vi "Rename Category.vi"(8 "error in (no error)":errorcluster, 9 "New Name":string, 10 "Old Name":string, 11 "Budgetizer in":refnum<class "Budgetizer.lvclass">) -> (0 "error out":errorcluster, 2 "Anything Renamed?":bool, 3 "Budgetizer out":refnum<class "Budgetizer.lvclass">)   [LabVIEW 2018, in "Budgetizer.lvclass"]
uses:
  Budgetizer.lvclass
  Budgetizer.lvclass/Budgetizer.ctl
  database/Database.lvclass
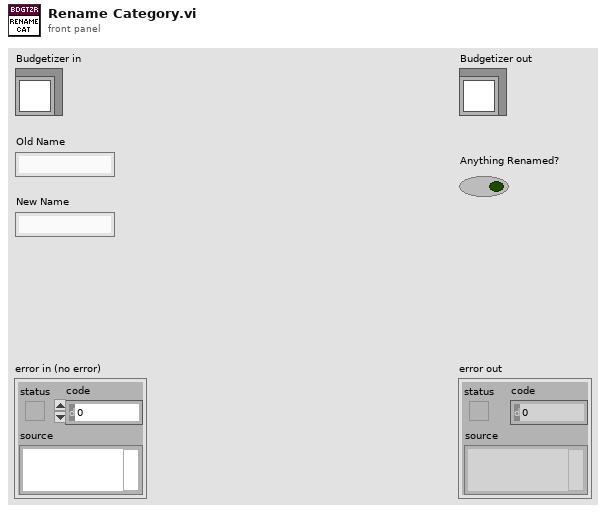
[diagram p1: front panel]
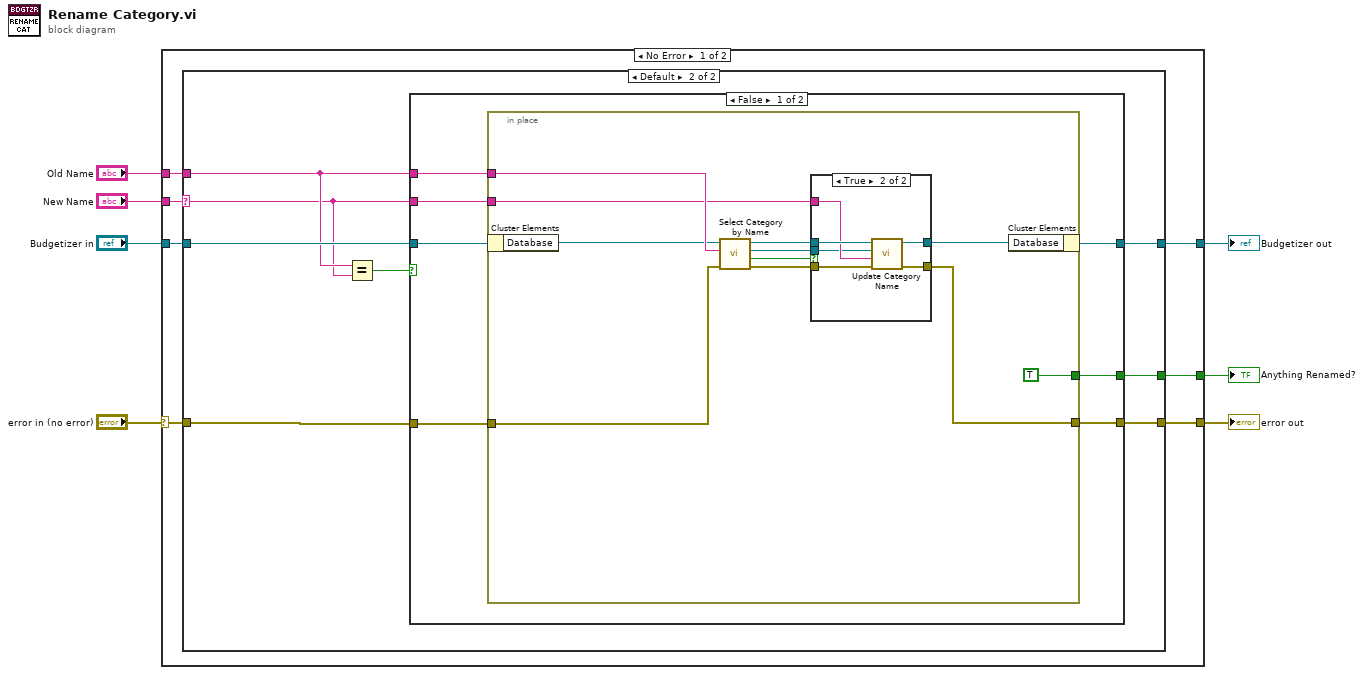
[diagram p0: block diagram]
diagram:
  n1 = case shown="No Error" "error in (no error)" {
    selector: "error in (no error)" -> [w9 w54]
    tunnel: [w8 w54] -> w6
    tunnel: [w10 w53] -> w4
    tunnel: "Budgetizer in" -> [w12 w53]
    tunnel: "Old Name" -> [w14 _]
    tunnel: "New Name" -> [w11 _]
    tunnel: [w13 _] -> w1
    frame No Error {
      n2 = case shown="Default" w11 {
        selector: w11 -> [_ w18]
        tunnel: w14 -> [_ w19]
        tunnel: [_ w20] -> w13
        tunnel: w12 -> [w16 w23]
        tunnel: [w16 w22] -> w10
        tunnel: w9 -> [w15 w24]
        tunnel: [w15 w21] -> w8
        frame "" {
        }
        frame Default {
          n3 = Equal?(x=w19, y=w18) -> (x = y?=w17:bool)
          n4 = case shown="False" w17 {
            tunnel: w24 -> [w28 w52]
            tunnel: w23 -> [w31 w51]
            tunnel: [w30 w51] -> w22
            tunnel: w19 -> [w29 _]
            tunnel: w18 -> [w27 _]
            tunnel: [w26 w52] -> w21
            tunnel: [w25 _] -> w20
            frame False {
              n5 = in-place {
                in-place-border: w29 -> [w41]
                in-place-border: w28 -> [w39]
                in-place-border: w27 -> [w36]
                in-place-border: [w34] -> w26
                in-place-border: [TRUE ("Anything Deleted?")] -> w25
                n6 = in-place-cluster #1(w31) -> ("Database"=w40:refnum<class "Database.lvclass">)
                n7 = call "Select Category by Name.vi"("error in (no error)"=w39, "Category Name"=w41, "Database in"=w40) -> ("error out"=w35:errorcluster, "Found?"=w32:bool, "Category"=w33:refnum<class "Category.lvclass">, "Database out"=w38:refnum<class "Database.lvclass">)  [unwired: 5 in]
                n8 = case shown="True" w32 {
                  tunnel: w38 -> [w44 w50]
                  tunnel: [w44 w49] -> w37
                  tunnel: w36 -> [_ w48]
                  tunnel: w35 -> [w43 w47]
                  tunnel: [w43 w46] -> w34
                  tunnel: w33 -> [_ w45]
                  frame False {
                  }
                  frame True {
                    n9 = call "Update Category Name.vi"("error in (no error)"=w47, "Name"=w48, "Category in"=w45, "Database in"=w50) -> ("error out"=w46:errorcluster, "Database out"=w49:refnum<class "Database.lvclass">)  [unwired: 6 in]
                  }
                }
                n10 = in-place-cluster #1("Database"=w37) -> (w30:refnum<class "Budgetizer.lvclass">)
              }
            }
            frame True {
            }
          }
        }
      }
    }
    frame Error {
    }
  }
  "error out" <- w6
  "Budgetizer out" <- w4
  "Anything Renamed?" <- w1
